vi "Find Next Galvo Input (SubVI).vi"(5 "Y Reverse":bool, 7 "X Reverse":bool, 8 "Deviation":cluster{"X":i32, "Y":i32}, 11 "Current GALVO Voltage":cluster{"X":dbl, "Y ":dbl} {"X" format="%.3f"; "Y" format="%.3f"}) -> (0 "Target Spot Reached?":bool, 3 "Next GALVO Volage":cluster{"X":dbl, "Y ":dbl} {"X" format="%.3f"; "Y" format="%.3f"})   [LabVIEW 2017]
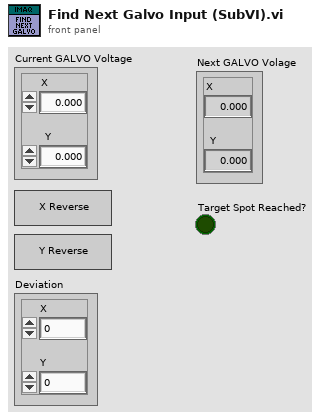
[diagram p1: front panel]
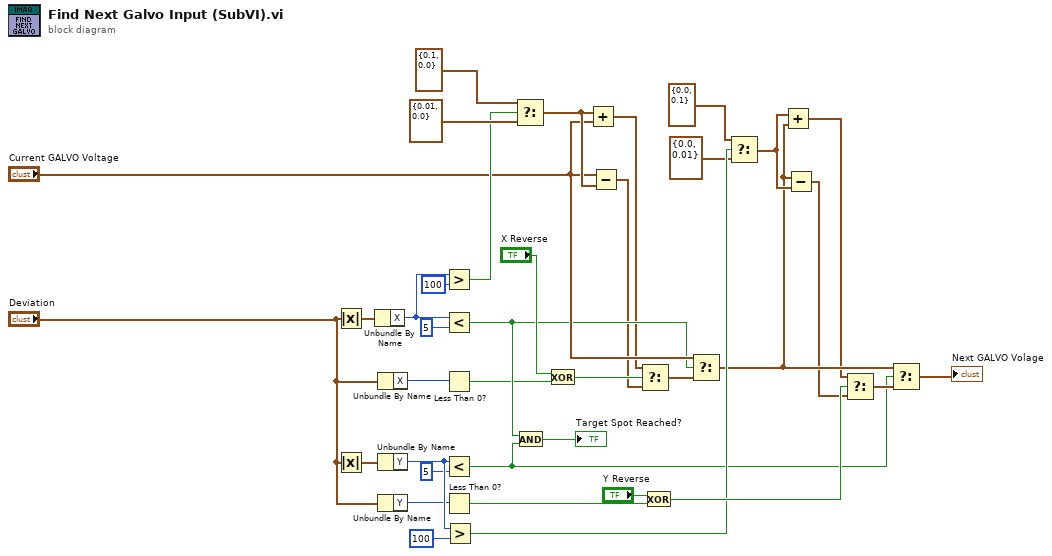
[diagram p0: block diagram]
diagram:
  n1 = Absolute Value(x="Deviation") -> (abs(x)=w27:cluster{"X":i32, "Y":i32})
  n2 = Absolute Value(x="Deviation") -> (abs(x)=w30:cluster{"X":i32, "Y":i32})
  n3 = Unbundle By Name(w27) -> ("X"=w35:i32)
  n4 = Unbundle By Name("Deviation") -> ("X"=w31:i32)
  n5 = Unbundle By Name(w30) -> ("Y"=w36:i32)
  n6 = Unbundle By Name("Deviation") -> ("Y"=w34:i32)
  n7 = Greater?(x=w35, y=100) -> (0:w16:bool)
  n8 = Less?(x=w35, y=5) -> (x < y?=w5:bool)
  n9 = Less Than 0?(x=w31) -> (x < 0?=w1:bool)
  n10 = Less?(x=w36, y=5) -> (x < y?=w9:bool)
  n11 = Less Than 0?(x=w34) -> (x < 0?=w14:bool)
  n12 = Greater?(x=w36, y=100) -> (0:w22:bool)
  n13 = Select(t=cluster{"X":dbl, "Y ":dbl} {"X"=0.1, "Y "=0.0} ("x"), s=w16, f=cluster{"X":dbl, "Y ":dbl} {"X"=0.01, "Y "=0.0} ("x")) -> (s? t:f=w17:cluster{"X":dbl, "Y ":dbl})
  n14 = And(x=w5, y=w9) -> (x .and. y?=→"Target Spot Reached?":bool)
  n15 = Exclusive Or(1:w1, 2:"X Reverse") -> (0:w23:bool)
  n16 = Add(x=w17, y="Current GALVO Voltage") -> (x+y=w3:cluster{"X":dbl, "Y ":dbl})
  n17 = Subtract(x="Current GALVO Voltage", y=w17) -> (x-y=w2:cluster{"X":dbl, "Y ":dbl})
  n18 = Select(t=w3, s=w23, f=w2) -> (s? t:f=w4:cluster{"X":dbl, "Y ":dbl})
  n19 = Exclusive Or(1:w14, 2:"Y Reverse") -> (0:w24:bool)
  n20 = Select(t="Current GALVO Voltage", s=w5, f=w4) -> (s? t:f=w13:cluster{"X":dbl, "Y ":dbl})
  n21 = Select(t=cluster{"X":dbl, "Y ":dbl} {"X"=0.0, "Y "=0.1} ("x"), s=w22, f=cluster{"X":dbl, "Y ":dbl} {"X"=0.0, "Y "=0.01} ("x")) -> (s? t:f=w19:cluster{"X":dbl, "Y ":dbl})
  n22 = Add(x=w19, y=w13) -> (x+y=w11:cluster{"X":dbl, "Y ":dbl})
  n23 = Subtract(x=w13, y=w19) -> (x-y=w12:cluster{"X":dbl, "Y ":dbl})
  n24 = Select(t=w11, s=w24, f=w12) -> (s? t:f=w10:cluster{"X":dbl, "Y ":dbl})
  n25 = Select(t=w13, s=w9, f=w10) -> (s? t:f=→"Next GALVO Volage":cluster{"X":dbl, "Y ":dbl})
